vi "h5_write_UTC_timestamp.vi"(7 "object name":string, 8 "error in (no error)":errorcluster, 10 "tiemsamp":timestamp caption="tiemsamp (now)", 11 "h5 obj ref":T1 format="%.0x") -> (0 "error out":errorcluster, 3 "h5 obj ref":T1 format="%.0x")   [LabVIEW 2015]
uses:
  <vilib>/addons/h5labview2/base/hid_t.ctl
  timing_tools/polys/poly_now_date_time.vi
  <vilib>/addons/h5labview2/base/lib_path.vi
  <vilib>/addons/h5labview2/base/H5Equery.vi
  <vilib>/addons/h5labview2/attrib/H5Awrite.llb/H5Awrite.xnode
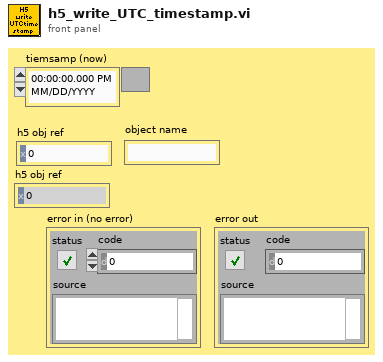
[diagram p1: front panel]
types:
  T1 = typedef "hid_t.ctl" = i32
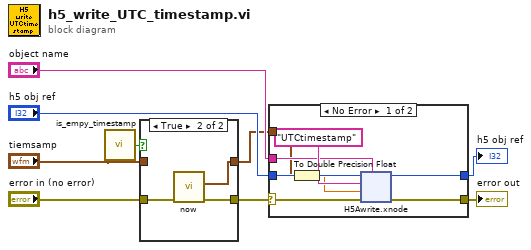
[diagram p0: block diagram]
diagram:
  n1 = call "is_empy_timestamp.vi"("time stamp"="tiemsamp") -> ("is empty?"=w5:bool)  [unwired: 8 in]
  n2 = case shown="True" w5 {
    tunnel: [w11 w14] -> w4
    tunnel: "tiemsamp" -> [w11 _]
    tunnel: "error in (no error)" -> [w10 w13]
    tunnel: [w10 w12] -> w1
    frame False {
    }
    frame True {
      n3 = call-poly "now.vi"("Error in"=w13) -> ("Error out"=w12:errorcluster, "current time"=w14:timestamp)  [unwired: 9 in]
    }
  }
  n4 = case shown="No Error" w1 {
    selector: w1 -> [w17 w43]
    tunnel: "object name" -> [w21 _]
    tunnel: [w20 w43] -> w9
    tunnel: [w19 w42] -> w6
    tunnel: "h5 obj ref" -> [w18 w42]
    tunnel: w4 -> [w16 _]
    frame No Error {
      n5 = To Double Precision Float(number=w16) -> (double precision float=w15:dbl)
      n6 = xnode "H5Awrite.xnode"("object name"=w21, "error in (no error)"=w17, "data"=w15, "attrib name"="UTCtimestamp", "ref in"=w18) -> ("error out"=w20:errorcluster, "ref out"=w19:i32)  [unwired: 2 in, 1 out]
    }
    frame Error {
    }
  }
  "error out" <- w9
  "h5 obj ref" <- w6
